vi "IntanInit.vi"(8 "error in (no error)":errorcluster, 11 "IntanElectrophysiology in":refnum<class "IntanElectrophysiology.lvclass">) -> (0 "error out":errorcluster, 3 "IntanElectrophysiology out":refnum<class "IntanElectrophysiology.lvclass">)   [LabVIEW 2014, in "IntanElectrophysiology.lvclass"]
uses:
  IntanElectrophysiology.lvclass
  IntanElectrophysiology.lvclass/IntanElectrophysiology.ctl
panel:
  in  "Intan Board Error":errorcluster
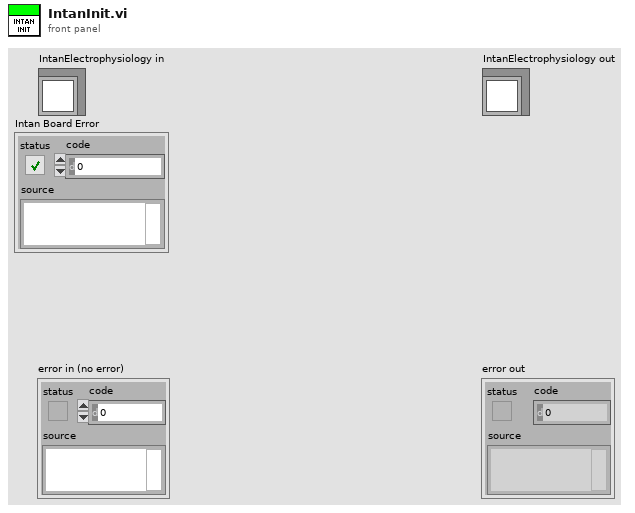
[diagram p1: front panel]
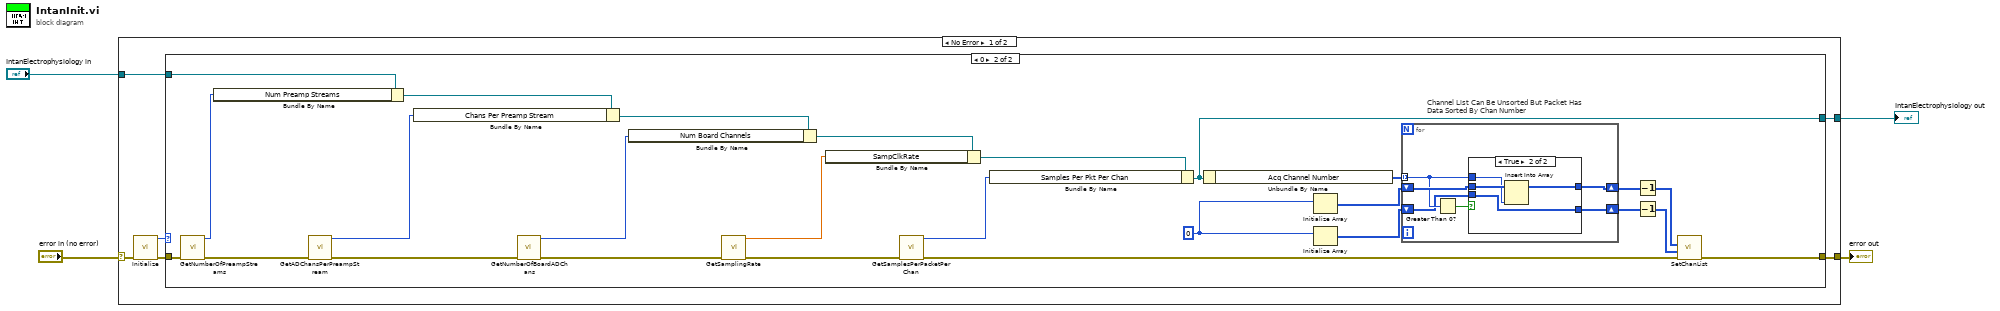
[diagram p0: block diagram]
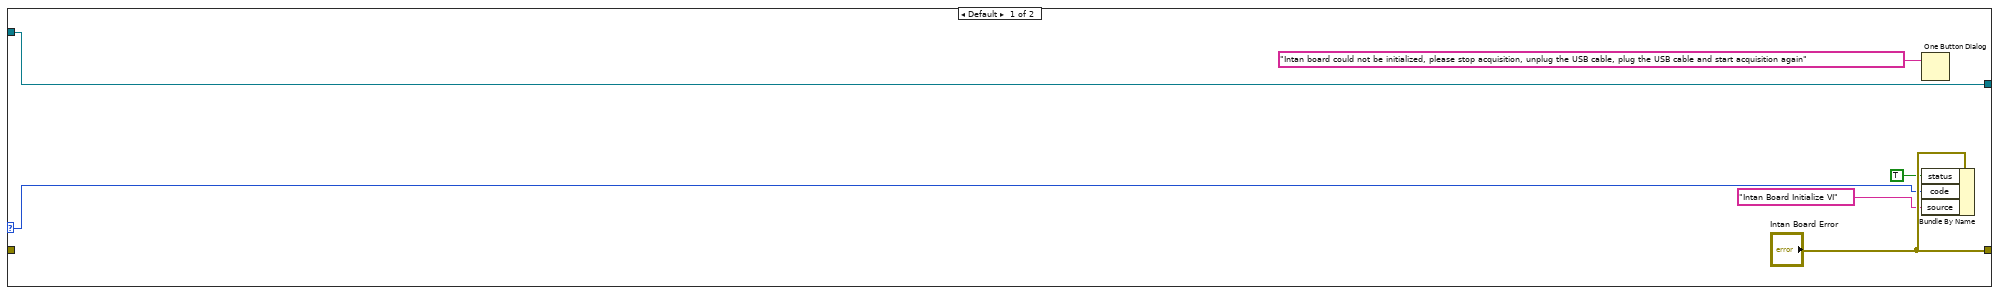
[diagram p2: hidden frame]
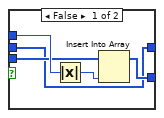
[diagram p3: hidden frame]
diagram:
  n1 = case shown="No Error" "error in (no error)" {
    selector: "error in (no error)" -> [w9 w59]
    tunnel: [w8 w59] -> w3
    tunnel: [w7 w58] -> w1
    tunnel: "IntanElectrophysiology in" -> [w6 w58]
    frame No Error {
      n2 = call "Initialize.vi"("error in (no error)"=w9) -> ("error out"=w10:errorcluster, "Return"=w5:i32)  [unwired: 9 in]
      n3 = case shown="0" w5 {
        selector: w5 -> [w13 _]
        tunnel: w10 -> [_ w42]
        tunnel: ["Intan Board Error" w17] -> w8
        tunnel: [w16 w26] -> w7
        tunnel: w6 -> [w16 w31]
        frame Default {
          n4 = One Button Dialog(message="Intan board could not be initialized, please stop acquisition, unplug the USB cable, plug the USB cable and start acquisition again") -> ()  [unwired: 1 in, 1 out]
          n5 = Bundle By Name(cluster="Intan Board Error", "status"=TRUE, "code"=w13, "source"="Intan Board Initialize VI") -> ()  [unwired: 1 out]
        }
        frame 0 {
          w27 = 0 ("element")
          n6 = call "GetNumberOfPreampStreams.vi"("error in (no error)"=w42) -> ("error out"=w40:errorcluster, "Return"=w41:i32)  [unwired: 9 in]
          n7 = Bundle By Name(cluster=w31, "Num Preamp Streams"=w41) -> (w30:refnum<class "IntanElectrophysiology.lvclass">)
          n8 = call "GetADChansPerPreampStream.vi"("error in (no error)"=w40) -> ("error out"=w38:errorcluster, "Return"=w39:i32)  [unwired: 9 in]
          n9 = Bundle By Name(cluster=w30, "Chans Per Preamp Stream"=w39) -> (w29:refnum<class "IntanElectrophysiology.lvclass">)
          n10 = call "GetNumberOfBoardADChans.vi"("error in (no error)"=w38) -> ("error out"=w36:errorcluster, "Return"=w37:i32)  [unwired: 9 in]
          n11 = Bundle By Name(cluster=w29, "Num Board Channels"=w37) -> (w28:refnum<class "IntanElectrophysiology.lvclass">)
          n12 = call "GetSamplingRate.vi"("error in (no error)"=w36) -> ("error out"=w34:errorcluster, "Return"=w35:dbl)  [unwired: 9 in]
          n13 = Bundle By Name(cluster=w28, "SampClkRate"=w35) -> (w32:refnum<class "IntanElectrophysiology.lvclass">)
          n14 = call "GetSamplesPerPacketPerChan.vi"("error in (no error)"=w34) -> ("error out"=w18:errorcluster, "Return"=w33:i32)  [unwired: 9 in]
          n15 = Bundle By Name(cluster=w32, "Samples Per Pkt Per Chan"=w33) -> (w26:refnum<class "IntanElectrophysiology.lvclass">)
          n16 = Unbundle By Name(w26) -> ("Acq Channel Number"=w25:i32[])
          n17 = Initialize Array(w27) -> (w24:i32[])  [unwired: 1 in]
          n18 = Initialize Array(w27) -> (w23:i32[])  [unwired: 1 in]
          n19 = for "Channel List Can Be Unsorted But Packet Has Data Sorted By Chan Number" {
            tunnel: w25 -> [w46] mode=indexing
            shift-right: [w43] -> w22
            shift-left: w24 -> [w47]
            shift-right: [w44] -> w21
            shift-left: w23 -> [w45]
            n20 = Greater Than 0?(x=w46) -> (x > 0?=w48:bool)
            n21 = case shown="True" w48 {
              tunnel: w47 -> [w49 w56]
              tunnel: w46 -> [w53 w55]
              tunnel: [w50 w57] -> w44
              tunnel: w45 -> [w51 w57]
              tunnel: [w49 w54] -> w43
              frame False {
                n22 = Absolute Value(x=w53) -> (abs(x)=w52:i32)
                n23 = Insert Into Array(array=w51, new element=w52) -> (w50:i32[])  [unwired: 1 in]
              }
              frame True {
                n24 = Insert Into Array(array=w56, new element=w55) -> (w54:i32[])  [unwired: 1 in]
              }
            }
          }
          n25 = Decrement(x=w22) -> (x-1=w20:i32[])
          n26 = Decrement(x=w21) -> (x-1=w19:i32[])
          n27 = call "SetChanList.vi"("error in (no error)"=w18, "Board Amp List"=w19, "Preamp Chan List"=w20) -> ("error out"=w17:errorcluster)  [unwired: 7 in, 1 out]
        }
      }
    }
    frame Error {
    }
  }
  "error out" <- w3
  "IntanElectrophysiology out" <- w1
